vi "make xy voltage map.vi"() -> ()   [LabVIEW 2017]
doc: "SciScan 1.2 160622"
uses:
  GFG/GFGnumericGet.vi
  GFG/GFGbooleanGet.vi
  GFG/GFG library.lvlib
panel:
  out "x voltage":T1(plugin-control)
  out "y voltage":T1(plugin-control)
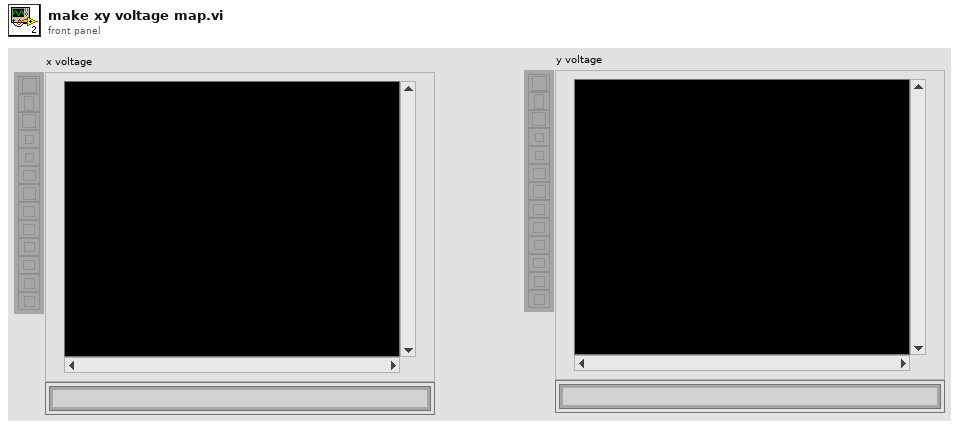
[diagram p1: front panel]
types:
  T1 = typedef "IMAQ Image.ctl" = refnum<image>
  T2 = cluster{"xyvoltagefor2frames":dbl[][][], "x.pixels":dbl, "nomin.x.pixels":dbl, "y.pixels":dbl, "fill.fraction":dbl, "x.bidirectional":bool, "y.bidirectional":bool}
  T3 = typedef "Image Type" = u32
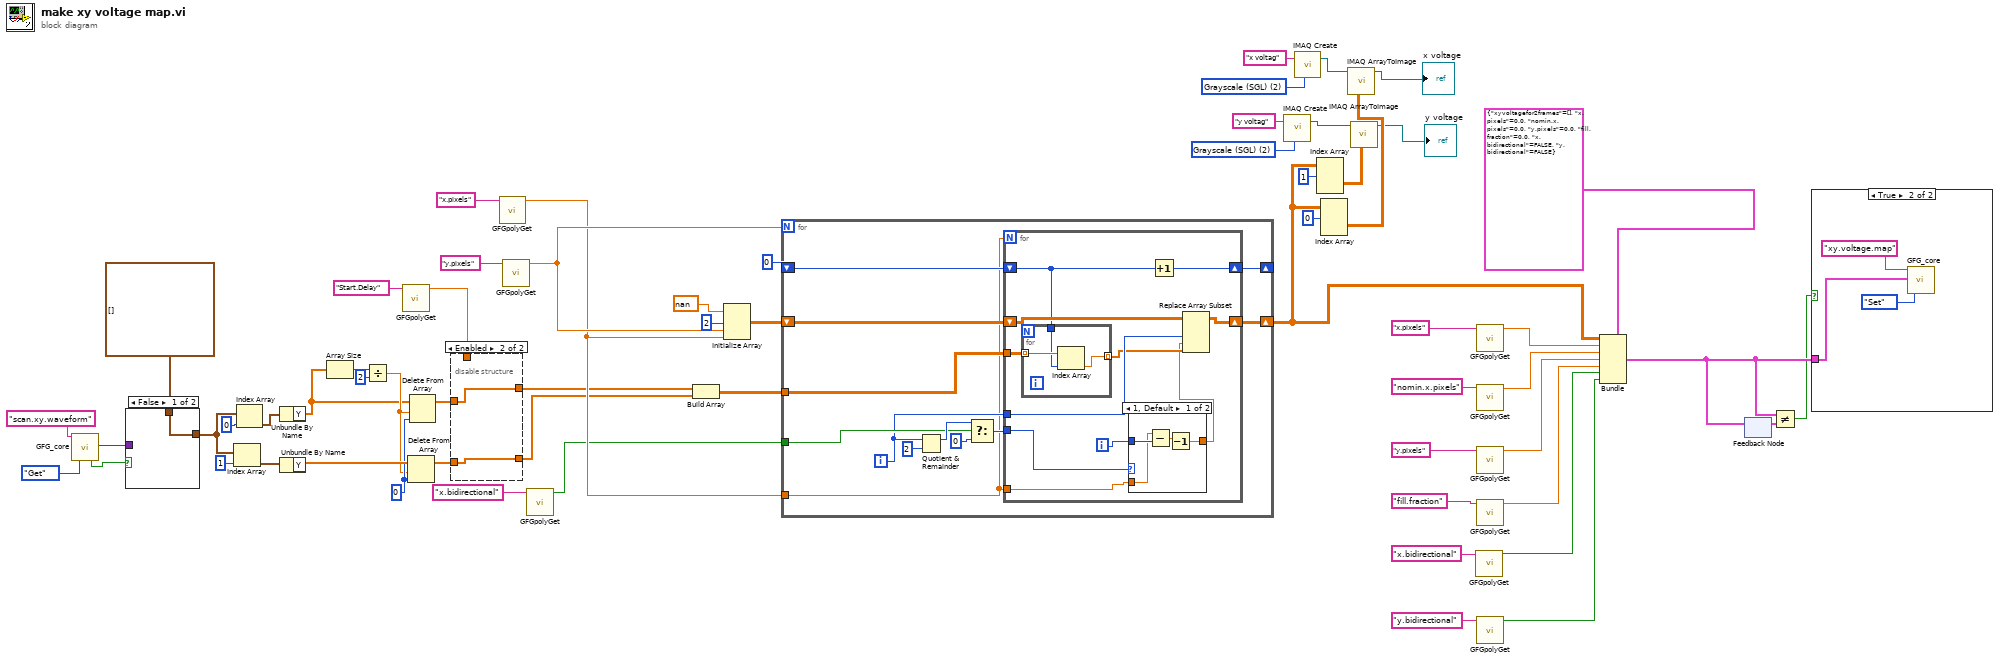
[diagram p0: block diagram]
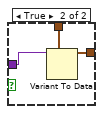
[diagram p2: hidden frame]
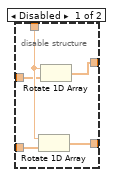
[diagram p4: hidden frame]
diagram:
  w27 = T3 2 items=["Grayscale (U8)", "Grayscale (I16)", "Grayscale (SGL)", "Complex (CSG)", "RGB (U32)", "HSL (U32)", "RGB (U64)", "Grayscale (U16)"] ("Image Type")
  w30 = T3 2 items=["Grayscale (U8)", "Grayscale (I16)", "Grayscale (SGL)", "Complex (CSG)", "RGB (U32)", "HSL (U32)", "RGB (U64)", "Grayscale (U16)"] ("Image Type")
  w44 = 0 ("index")
  n1 = call "GFG_core.vi"("Variable Name in"="scan.xy.waveform", "Action"=enum16{"Init", "Set", "Get"}."Get") -> ("Found/Replaced"=w1:bool, "Variant Out"=w33:variant)  [unwired: 11 in, 5 out]
  n2 = case shown="False" w1 {
    tunnel: [w63 w66] -> w35
    tunnel: waveform(dbl)[] [] ("frame scan geometry out") -> [w63 w65]
    tunnel: w33 -> [_ w64]
    frame False {
    }
    frame True {
      n3 = Variant To Data(type=w65, Variant=w64) -> (data=w66:waveform(dbl)[])  [unwired: 1 in, 1 out]
    }
  }
  n4 = Index Array(array=w35, index=1) -> (element=w39:waveform(dbl))
  n5 = Index Array(array=w35, index=0) -> (element=w38:waveform(dbl))
  n6 = Unbundle By Name(w38) -> ("Y"=w42:dbl[])
  n7 = Unbundle By Name(w39) -> ("Y"=w45:dbl[])
  n8 = Array Size(array=w42) -> (size(s)=w40:i32)
  n9 = Divide(x=w40, y=2) -> (x/y=w43:dbl)
  n10 = call-poly "GFGpolyGet.vi"("Variable Name in"="Start.Delay") -> ("Numeric"=w49:dbl)  [unwired: 8 in, 2 out]
  n11 = Delete From Array(array=w45, length=w43, index=w44) -> (array with subset deleted=w48:dbl[])  [unwired: 1 out]
  n12 = Delete From Array(array=w42, length=w43, index=w44) -> (array with subset deleted=w46:dbl[])  [unwired: 1 out]
  n13 = disable-structure shown="Enabled" {
    disable-tunnel: [w71 w72] -> w58
    disable-tunnel: [w70 w73] -> w57
    disable-tunnel: w49 -> [w69 _]
    disable-tunnel: w48 -> [w68 w72]
    disable-tunnel: w46 -> [w67 w73]
    frame Disabled {
      n14 = Rotate 1D Array(1:w68, 2:w69) -> (0:w71:dbl[])
      n15 = Rotate 1D Array(1:w67, 2:w69) -> (0:w70:dbl[])
    }
    frame Enabled {
    }
  }
  n16 = call-poly "GFGpolyGet.vi"("Variable Name in"="x.pixels" ("Tag in")) -> ("Numeric"=w60:dbl)  [unwired: 8 in, 2 out]
  n17 = call-poly "GFGpolyGet.vi"("Variable Name in"="y.pixels" ("Tag in")) -> ("Numeric"=w61:dbl)  [unwired: 8 in, 2 out]
  n18 = call-poly "GFGpolyGet.vi"("Variable Name in"="x.bidirectional" ("Tag in")) -> ("Boolean Value OUT"=w53:bool)  [unwired: 9 in, 1 out]
  n19 = Build Array(w57, w58) -> (w59:dbl[][])
  n20 = Initialize Array(nan ("element"), 2 ("dimension size"), w61, w60) -> (w55:dbl[][][])
  n21 = for {
    N: w61 -> [_]
    tunnel: w60 -> [w75]
    tunnel: w53 -> [w81]
    shift-right: [w74] -> w8
    shift-left: w55 -> [w78]
    shift-right: [w79] -> _
    shift-left: 0 ("y") -> [w80]
    tunnel: w59 -> [w76]
    i -> [w77]
    n22 = Quotient & Remainder(x=w77, y=2) -> (x-y*floor(x/y)=w85:i32)  [unwired: 1 out]
    n23 = Select(t=w85, s=w81, f=0) -> (s? t:f=w82:i32)
    n24 = for {
      N: w75 -> [_]
      tunnel: w82 -> [w96]
      shift-right: [w95] -> w79
      shift-left: w80 -> [w88]
      shift-right: [w92] -> w74
      shift-left: w78 -> [w93]
      tunnel: w77 -> [w91]
      tunnel: w76 -> [w90]
      tunnel: w75 -> [w86]
      i -> [w94]
      n25 = for {
        tunnel: w90 -> [w99] mode=indexing
        tunnel: w88 -> [w98]
        tunnel: [w97] -> w89 mode=indexing
        n26 = Index Array(array=w99, index=w98) -> (element=w97:dbl)
      }
      n27 = case shown="1, Default" w96 {
        tunnel: w94 -> [w103 w104]
        tunnel: [w100 w104] -> w87
        tunnel: w86 -> [w102 _]
        frame 1, Default {
          n28 = Subtract(x=w102, y=w103) -> (x-y=w101:dbl)
          n29 = Decrement(x=w101) -> (x-1=w100:dbl)
        }
        frame 0 {
        }
      }
      n30 = Increment(x=w88) -> (x+1=w95:i32)
      n31 = Replace Array Subset(array=w93, new element=w89, index (dim 1)=w91, index (dim 2)=w87) -> (w92:dbl[][][])  [unwired: 1 in]
    }
  }
  n32 = call "IMAQ Create"("Image Name"="y voltag", "Image Type"=w27) -> ("New Image"=w25:T1)  [unwired: 3 in, 1 out]
  n33 = call "IMAQ Create"("Image Name"="x voltag", "Image Type"=w30) -> ("New Image"=w26:T1)  [unwired: 3 in, 1 out]
  n34 = Index Array(array=w8, index (dim 0)=1 ("index (page)")) -> (element=w20:dbl[][])  [unwired: 2 in]
  n35 = Index Array(array=w8, index (dim 0)=0 ("index (page)")) -> (element=w23:dbl[][])  [unwired: 2 in]
  n36 = call "IMAQ ArrayToImage"("Image Pixels (Float)"=w23, "Image"=w26) -> ("Image Out"=→"x voltage":T1)  [unwired: 8 in, 1 out]
  n37 = call "IMAQ ArrayToImage"("Image Pixels (Float)"=w20, "Image"=w25) -> ("Image Out"=→"y voltage":T1)  [unwired: 8 in, 1 out]
  n38 = call-poly "GFGpolyGet.vi"("Variable Name in"="x.bidirectional" ("Tag in")) -> ("Boolean Value OUT"=w9:bool)  [unwired: 9 in, 1 out]
  n39 = call-poly "GFGpolyGet.vi"("Variable Name in"="x.pixels" ("Tag in")) -> ("Numeric"=w13:dbl)  [unwired: 8 in, 2 out]
  n40 = call-poly "GFGpolyGet.vi"("Variable Name in"="nomin.x.pixels") -> ("Numeric"=w12:dbl)  [unwired: 8 in, 2 out]
  n41 = call-poly "GFGpolyGet.vi"("Variable Name in"="y.pixels" ("Tag in")) -> ("Numeric"=w11:dbl)  [unwired: 8 in, 2 out]
  n42 = call-poly "GFGpolyGet.vi"("Variable Name in"="fill.fraction") -> ("Numeric"=w10:dbl)  [unwired: 8 in, 2 out]
  n43 = call-poly "GFGpolyGet.vi"("Variable Name in"="y.bidirectional" ("Tag in")) -> ("Boolean Value OUT"=w5:bool)  [unwired: 9 in, 1 out]
  n44 = Bundle(cluster=T2 {"xyvoltagefor2frames"=[], "x.pixels"=0.0, "nomin.x.pixels"=0.0, "y.pixels"=0.0, "fill.fraction"=0.0, "x.bidirectional"=FALSE, "y.bidirectional"=FALSE} ("output cluster"), "xyvoltagefor2frames"=w8, "x.pixels"=w13, "nomin.x.pixels"=w12, "y.pixels"=w11, "fill.fraction"=w10, "x.bidirectional"=w9, "y.bidirectional"=w5) -> (w3:T2)
  n45 = feedback #1() -> (w4:T2)  [unwired: 1 in]
  n46 = feedback-in #1(w3) -> ()
  n47 = Not Equal?(x=w3, y=w4) -> (x != y?=w2:bool)
  n48 = case shown="True" w2 {
    tunnel: w3 -> [_ w105]
    frame False {
    }
    frame True {
      n49 = call "GFG_core.vi"("Variable Name in"="xy.voltage.map", "Variant in"=w105, "Action"=enum16{"Init", "Set", "Get"}."Set") -> ()  [unwired: 10 in, 7 out]
    }
  }
